vi "Get Common Prefix or Suffix from String List.vi"(10 "Strings":string[](array[string])) -> (1 "Common Part":string, 2 "Suffix? (F: Prefix)":bool)   [LabVIEW 2009]
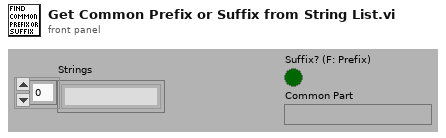
[diagram p1: front panel]
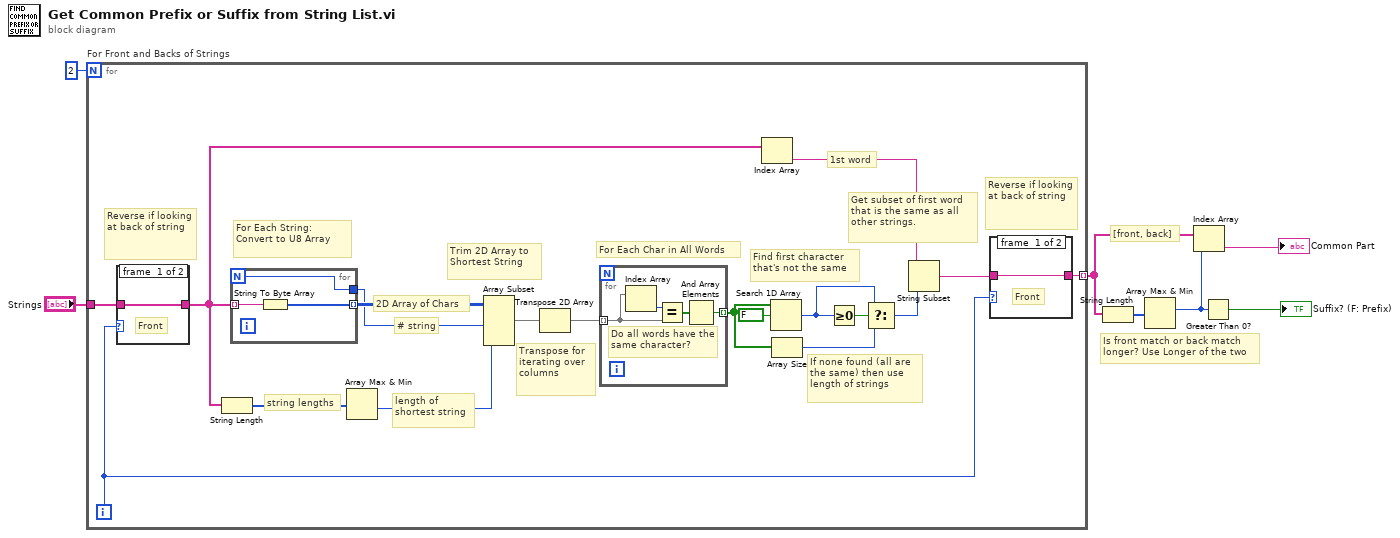
[diagram p0: block diagram]
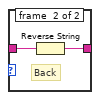
[diagram p2: hidden frame]
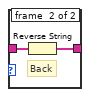
[diagram p3: hidden frame]
diagram:
  # "[front, back]"
  # "Is front match or back match longer? Use Longer of the two"
  n1 = for "For Front and Backs of Strings" {
    N: 2 -> [_]
    tunnel: "Strings" -> [w20]
    tunnel: [w12] -> w4 mode=indexing
    i -> [w11]
    # "For Each Char in All Words"
    # "For Each String: Convert to U8 Array"
    # "Reverse if looking at back of string"
    # "Reverse if looking at back of string"
    # "Get subset of first word that is the same as all other strings."
    # "1st word"
    # "If none found (all are the same) then use length of strings"
    # "Find first character that's not the same"
    # "Transpose for iterating over columns"
    # "Trim 2D Array to Shortest String"
    # "2D Array of Chars"
    # "# string"
    # "length of shortest string"
    # "string lengths"
    n2 = case shown="Default" w11 {
      tunnel: w20 -> [w29 w31]
      tunnel: [w29 w30] -> w9
      frame #0 {
        # "Front"
      }
      frame #1 {
        # "Back"
        n3 = Reverse String(1:w31) -> (0:w30:string[])
      }
    }
    n4 = String Length(string=w9) -> (length=w8:i32[])
    n5 = for {
      N -> [w36]
      tunnel: w9 -> [w38] mode=indexing
      tunnel: [w37] -> w18 mode=indexing
      tunnel: [w36] -> w17
      n6 = String To Byte Array(string=w38) -> (unsigned byte array=w37:u8[])
    }
    n7 = Array Max & Min(array=w8) -> (min value=w16:i32)  [unwired: 3 out]
    n8 = Array Subset(array=w18, length (row)=w17, length (col)=w16) -> (w15:u8[][])  [unwired: 2 in]
    n9 = Transpose 2D Array(2D array=w15) -> (transposed array=w19:u8[][])
    n10 = for {
      tunnel: w19 -> [w35] mode=indexing
      tunnel: [w32] -> w23 mode=indexing
      # "Do all words have the same character?"
      n11 = Index Array(array=w35) -> (element=w34:u8)  [unwired: 1 in]
      n12 = Equal?(x=w34, y=w35) -> (x = y?=w33:bool[])
      n13 = And Array Elements(Boolean array=w33) -> (logical AND=w32:bool)
    }
    n14 = Index Array(array=w9) -> (element=w10:string)  [unwired: 1 in]
    n15 = Search 1D Array(1D array=w23, element=FALSE) -> (index of element=w21:i32)  [unwired: 1 in]
    n16 = Array Size(array=w23) -> (size(s)=w22:i32)
    n17 = Greater Or Equal To 0?(x=w21) -> (x >= 0?=w24:bool)
    n18 = Select(t=w21, s=w24, f=w22) -> (s? t:f=w14:i32)
    n19 = String Subset(string=w10, length (rest)=w14) -> (substring=w13:string)  [unwired: 1 in]
    n20 = case shown="1" w11 {
      tunnel: w13 -> [w26 w28]
      tunnel: [w26 w27] -> w12
      frame #0 {
        # "Front"
      }
      frame #1 {
        # "Back"
        n21 = Reverse String(1:w28) -> (0:w27:string)
      }
    }
  }
  n22 = String Length(string=w4) -> (length=w6:i32[])
  n23 = Array Max & Min(array=w6) -> (max index (indices)=w3:i32)  [unwired: 3 out]
  n24 = Index Array(array=w4, index=w3) -> (element=→"Common Part":string)
  n25 = Greater Than 0?(x=w3) -> (x > 0?=→"Suffix? (F: Prefix)":bool)
